vi "Core Pre Launch Init.vi"(8 "error in (no error)":errorcluster, 11 "Instrument Sequencer in":refnum<class "Instrument Sequencer.lvclass">) -> (0 "error out":errorcluster, 3 "Instrument Sequencer out":refnum<class "Instrument Sequencer.lvclass">)   [LabVIEW 2020, in "Instrument Handler.lvlib" / "Instrument Sequencer.lvclass"]
doc: "This VI is executed during the Launch of the Sequencer Core. This will be executed during the Pre launch init phase of the Sequencer Actor.\n\nThis implementation initializes the Driver."
uses:
  Instrument Sequencer.lvclass
  Instrument Sequencer.lvclass/Instrument Sequencer.ctl
  PPL/HDH.Actor Framework.Core.Sequencer.lvlibp/Sequencer Core/Sequencer Core.lvclass
  PPL/HDH.Actor Framework.Core.Instrument Driver.lvlibp/Instrument Driver/Instrument Driver.lvclass
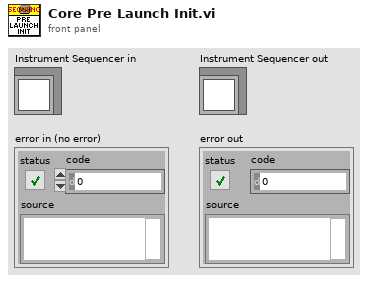
[diagram p1: front panel]
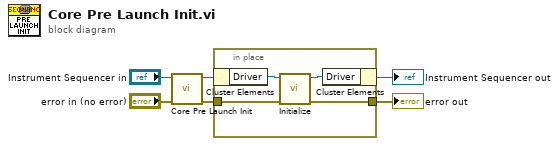
[diagram p0: block diagram]
diagram:
  n1 = call-parent "Core Pre Launch Init.vi"("error in (no error)"="error in (no error)", "Sequencer Core in"="Instrument Sequencer in") -> ("error out"=w3:errorcluster, "Sequencer Core out"=w1:refnum<class "Instrument Sequencer.lvclass">)  [unwired: 8 in]
  n2 = in-place {
    in-place-border: w3 -> [w8]
    in-place-border: [w7] -> w5
    n3 = in-place-cluster #1(w1) -> ("Driver"=w9:refnum<class "Instrument Driver.lvclass">)
    n4 = call "Initialize.vi"("error in (no error)"=w8, "Instrument in"=w9) -> ("error out"=w7:errorcluster, "Instrument out"=w10:refnum<class "Instrument Driver.lvclass">)  [unwired: 8 in]
    n5 = in-place-cluster #1("Driver"=w10) -> (→"Instrument Sequencer out":refnum<class "Instrument Sequencer.lvclass">)
  }
  "error out" <- w5
